vi "SUB-BLE Rx data (Mon)-ROM.vi"(5 "data in":u8[](array[numeric])) -> (1 "data Out":u8[](array[numeric]), 2 "Index":u8)   [LabVIEW 2015]
doc: "Use this template to create an application that executes repeatedly until you click the Stop button. This template polls the state of the Stop button and does not use events. Use the Top-Level Application template (not available in the Base package) to create a single-loop application with event handling."
panel:
  out "BLE Packet (buf)":u8[](array[numeric])
  out "BLE Packet (data)":u8[](array[numeric])
  # "ROM Data"
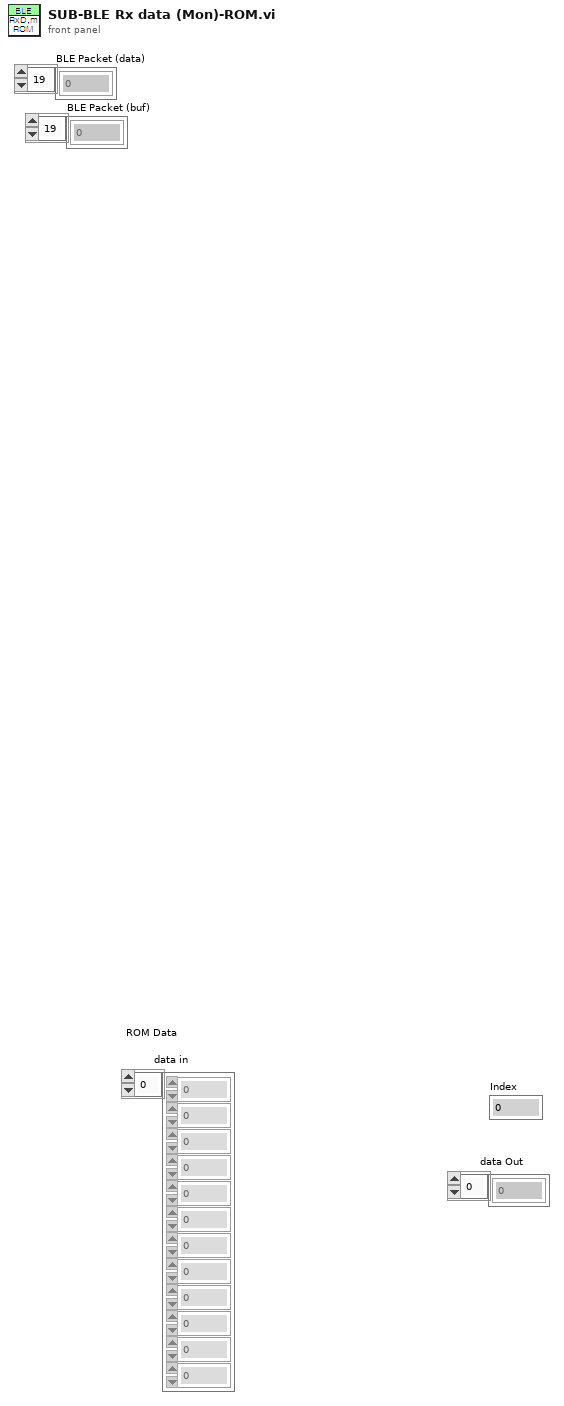
[diagram p1: front panel]
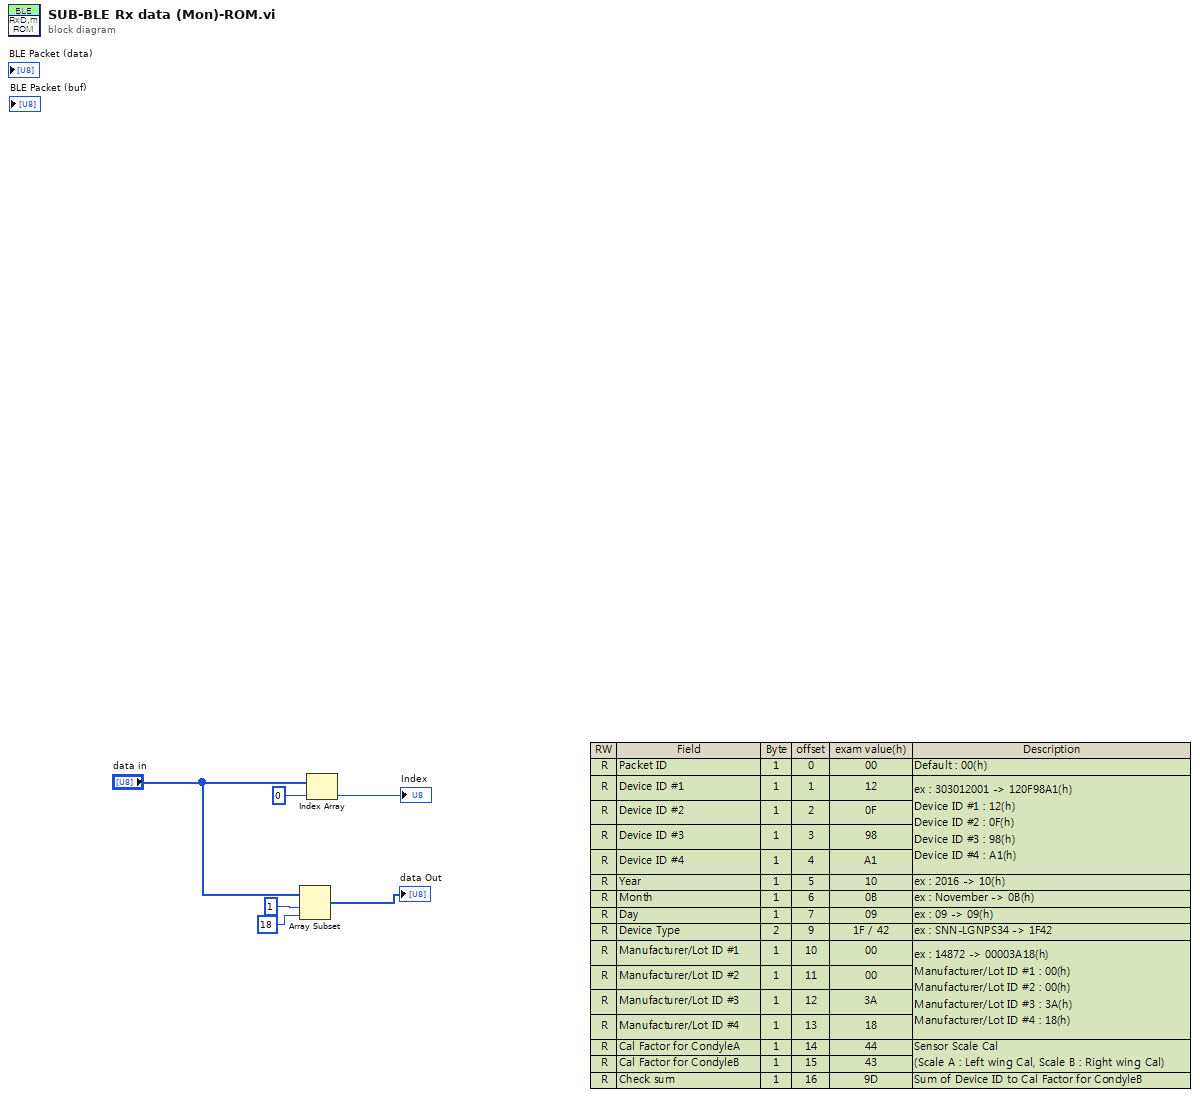
[diagram p0: block diagram]
diagram:
  n1 = Array Subset(array="data in", index=1 ("인덱스"), length=18 ("인덱스")) -> (→"data Out":u8[])
  n2 = Index Array(array="data in", index=0 ("인덱스")) -> (element=→"Index":u8)
